vi "Logging Smallest Unused Log Number.vi"(8 "error in (no error)":errorcluster, 9 "Starting Offset":i32, 10 "name":string="log", 11 "base path":path=path "c:/logs") -> (0 "error out":errorcluster, 1 "Number":i32, 2 "name out":string="log", 3 "base path out":path=path "c:/logs")   [LabVIEW 2012, in "femtoRoboLib.lvlib"]
uses:
  femtoRoboLib.lvlib
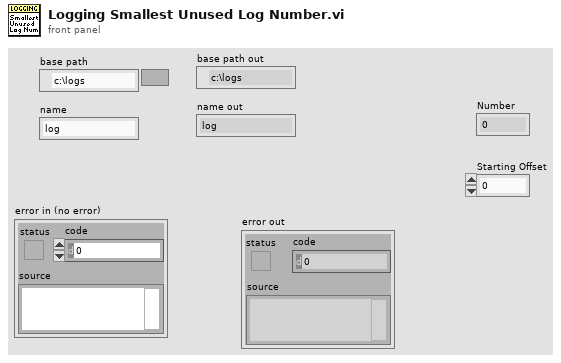
[diagram p1: front panel]
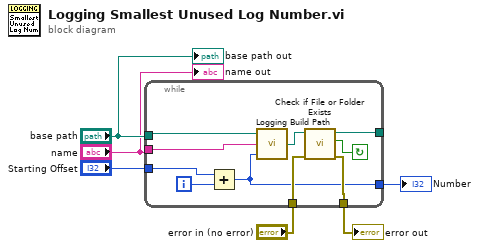
[diagram p0: block diagram]
diagram:
  n1 = while {
    tunnel: "base path" -> [w12]
    tunnel: [w16] -> _
    tunnel: "name" -> [w11]
    tunnel: "error in (no error)" -> [w14]
    tunnel: [w13] -> w5
    tunnel: [w8] -> w4
    tunnel: "Starting Offset" -> [w7]
    i -> [w10]
    stop <- w15 continue-if-true
    n2 = Add(x=w7, y=w10) -> (x+y=w8:i32)
    n3 = call "Logging Build Path.vi"("number"=w8, "name"=w11, "base path"=w12) -> ("built path"=w9:path)
    n4 = call <vilib>:"Check if File or Folder Exists.vi"("error in (no error)"=w14, "path"=w9) -> ("error out"=w13:errorcluster, "file or folder exists?"=w15:bool, "dup path"=w16:path)  [unwired: 7 in]
  }
  "error out" <- w5
  "Number" <- w4
  "base path out" <- "base path"
  "name out" <- "name"
